vi "wait.vi"(2 "error in":errorcluster, 3 "Wartezeit in Sek":dbl=1.0 format="%.2f") -> (0 "error out":errorcluster)   [LabVIEW 2010]
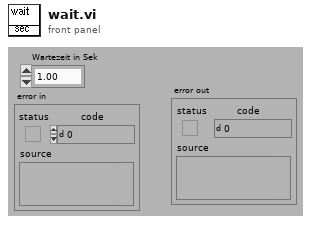
[diagram p1: front panel]
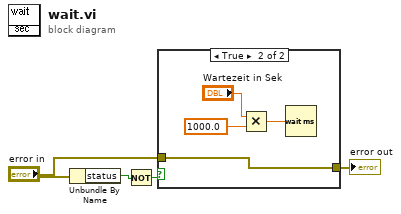
[diagram p0: block diagram]
diagram:
  n1 = Unbundle By Name("error in") -> ("status"=w3:bool)
  n2 = Not(x=w3) -> (.not. x?=w2:bool)
  n3 = case shown="True" w2 {
    tunnel: "error in" -> [w5 w6]
    tunnel: [w5 w6] -> w4
    frame False {
    }
    frame True {
      n4 = Multiply(x="Wartezeit in Sek", y=1000.0) -> (x*y=w7:dbl)
      n5 = Wait (ms)(milliseconds to wait=w7) -> ()  [unwired: 1 out]
    }
  }
  "error out" <- w4
